vi "Interp2D zp Demo.vi"(8 "XY Grid min":dbl[](array[numeric]), 9 "XY Quantization Factor":dbl[](array[numeric]), 10 "Zp array":dbl[][](array[numeric]), 11 "Tip Position":dbl[](array[numeric])) -> (3 "zp":dbl)   [LabVIEW 2016]
doc: "This VI takes in current (x,y) coordinate \"current x\" and \"current y\" and then output the distances to anterior capsule and posterior capsule based on 2D z data \"Zp array\" and \"Za array\" defined on a rectangular meshed grid (X,Y)..\nGiven current (x,y), zp and za distances are computed via 2D interpolation.\n\n\"index factor\" = (Xmax-Xmin)/size(sX) or (Ymax-Ymin)/size(Y)\n\"xy grid min\" = [Xmin Ymin]"
uses:
  Library/KevinLibraryAll/labview/KevLib01.lvlib
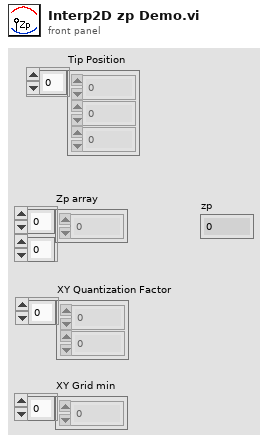
[diagram p1: front panel]
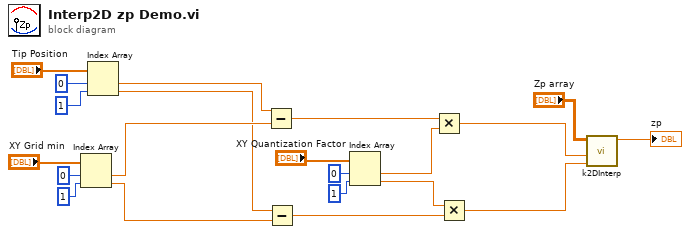
[diagram p0: block diagram]
diagram:
  n1 = Index Array(array="XY Grid min", index #1=0 ("index"), index #2=1 ("index")) -> (element #1=w17:dbl, element #2=w16:dbl)
  n2 = Index Array(array="Tip Position", index #1=0 ("index"), index #2=1 ("index")) -> (element #1=w8:dbl, element #2=w7:dbl)
  n3 = Subtract(x=w8, y=w17) -> (x-y=w15:dbl)
  n4 = Subtract(x=w7, y=w16) -> (x-y=w2:dbl)
  n5 = Index Array(array="XY Quantization Factor", index #1=0 ("index"), index #2=1 ("index")) -> (element #1=w3:dbl, element #2=w1:dbl)
  n6 = Multiply(x=w15, y=w3) -> (x*y=w14:dbl)
  n7 = Multiply(x=w1, y=w2) -> (x*y=w13:dbl)
  n8 = call "k2DInterp.vi"("col"=w13, "row"=w14, "Array"="Zp array") -> ("result"=→"zp":dbl)  [unwired: 8 in]
